vi "PID_position_radian.vi"() -> ()   [LabVIEW 2014]
uses:
  <vilib>/FPGAPlugInAG/cRIO-9068/niLvFpga_Open_cRIO-9068.vi
  <vilib>/rvi/interface/common/dynamic/niFpgaDynamicAddResources.vi
  <vilib>/Utility/error.llb/Error Cluster From Error Code.vi
  <vilib>/rvi/errors/niLvFpgaAdjustHostInterfaceError.vi
  <vilib>/addons/control/pid/pid.llb/PID (DBL).vi
  <vilib>/FPGAPlugInAG/Dynamic/niLvFpga_Close_Dynamic.vi
  <vilib>/rvi/interface/nirviOpenFPGA/nirviOpenFPGA.xnode
  FPGA Bitfiles/Motortest_FPGATarget_test6auto_Jx62XASY7Q8.lvbitx
  <vilib>/rvi/interface/nirviReadWriteControl/nirviReadWriteControl.xnode
  <vilib>/rvi/interface/nirviCloseFPGA/nirviCloseFPGA.xnode
  NiFpgaLv.dll
  <vilib>/rvi/interface/Simulation/niFpgaSimulationCallBeginRW.vi
  <vilib>/addons/control/pid/NI_PID_pid.lvlib
panel:
  in  "stop":bool
  out "Position [Round]":sgl
  out "Velocity [RPS]":sgl
  in  "PID Velocity":T1={"proportional gain (Kc)"=0.0006, "integral time (Ti, min)"=0.0005, "derivative time (Td, min)"=0.0} {"derivative time (Td, min)" format="%.4f"; "integral time (Ti, min)" format="%.4e"; "proportional gain (Kc)" format="%.4e"}
  in  "output range":cluster{"output high":dbl, "output low":dbl}={"output high"=1.0, "output low"=-1.0} {"output low" format="%.2f"; "output high" format="%.2f"}
  out "Velocity":sgl[](graph)
  out "Error":dbl(slide) scale=0.0..50.0
  out "Duty Cycle":dbl(slide) scale=0.0..1.0
  out "Duty Cycle 2":dbl[](graph)
  in  "Desired Position\n[Radian]":dbl=1500.0
  in  "PID Position":T1={"proportional gain (Kc)"=1.5, "integral time (Ti, min)"=0.0, "derivative time (Td, min)"=0.0} {"derivative time (Td, min)" format="%.3f"; "integral time (Ti, min)" format="%.3f"; "proportional gain (Kc)" format="%.3f"}
  out "Position":sgl[](graph)
  out "Velocity Setpoint":dbl[](graph)
  out "Velocity Setpoint [rad/second]":cluster{dbl[], dbl[]}(graph)
  out "Position [rad]":cluster{dbl[], sgl[]}(graph)
  out "Velocity [rad/second]":cluster{dbl[], sgl[]}(graph)
  out "Duty Cycle":cluster{dbl[], dbl[]}(graph)
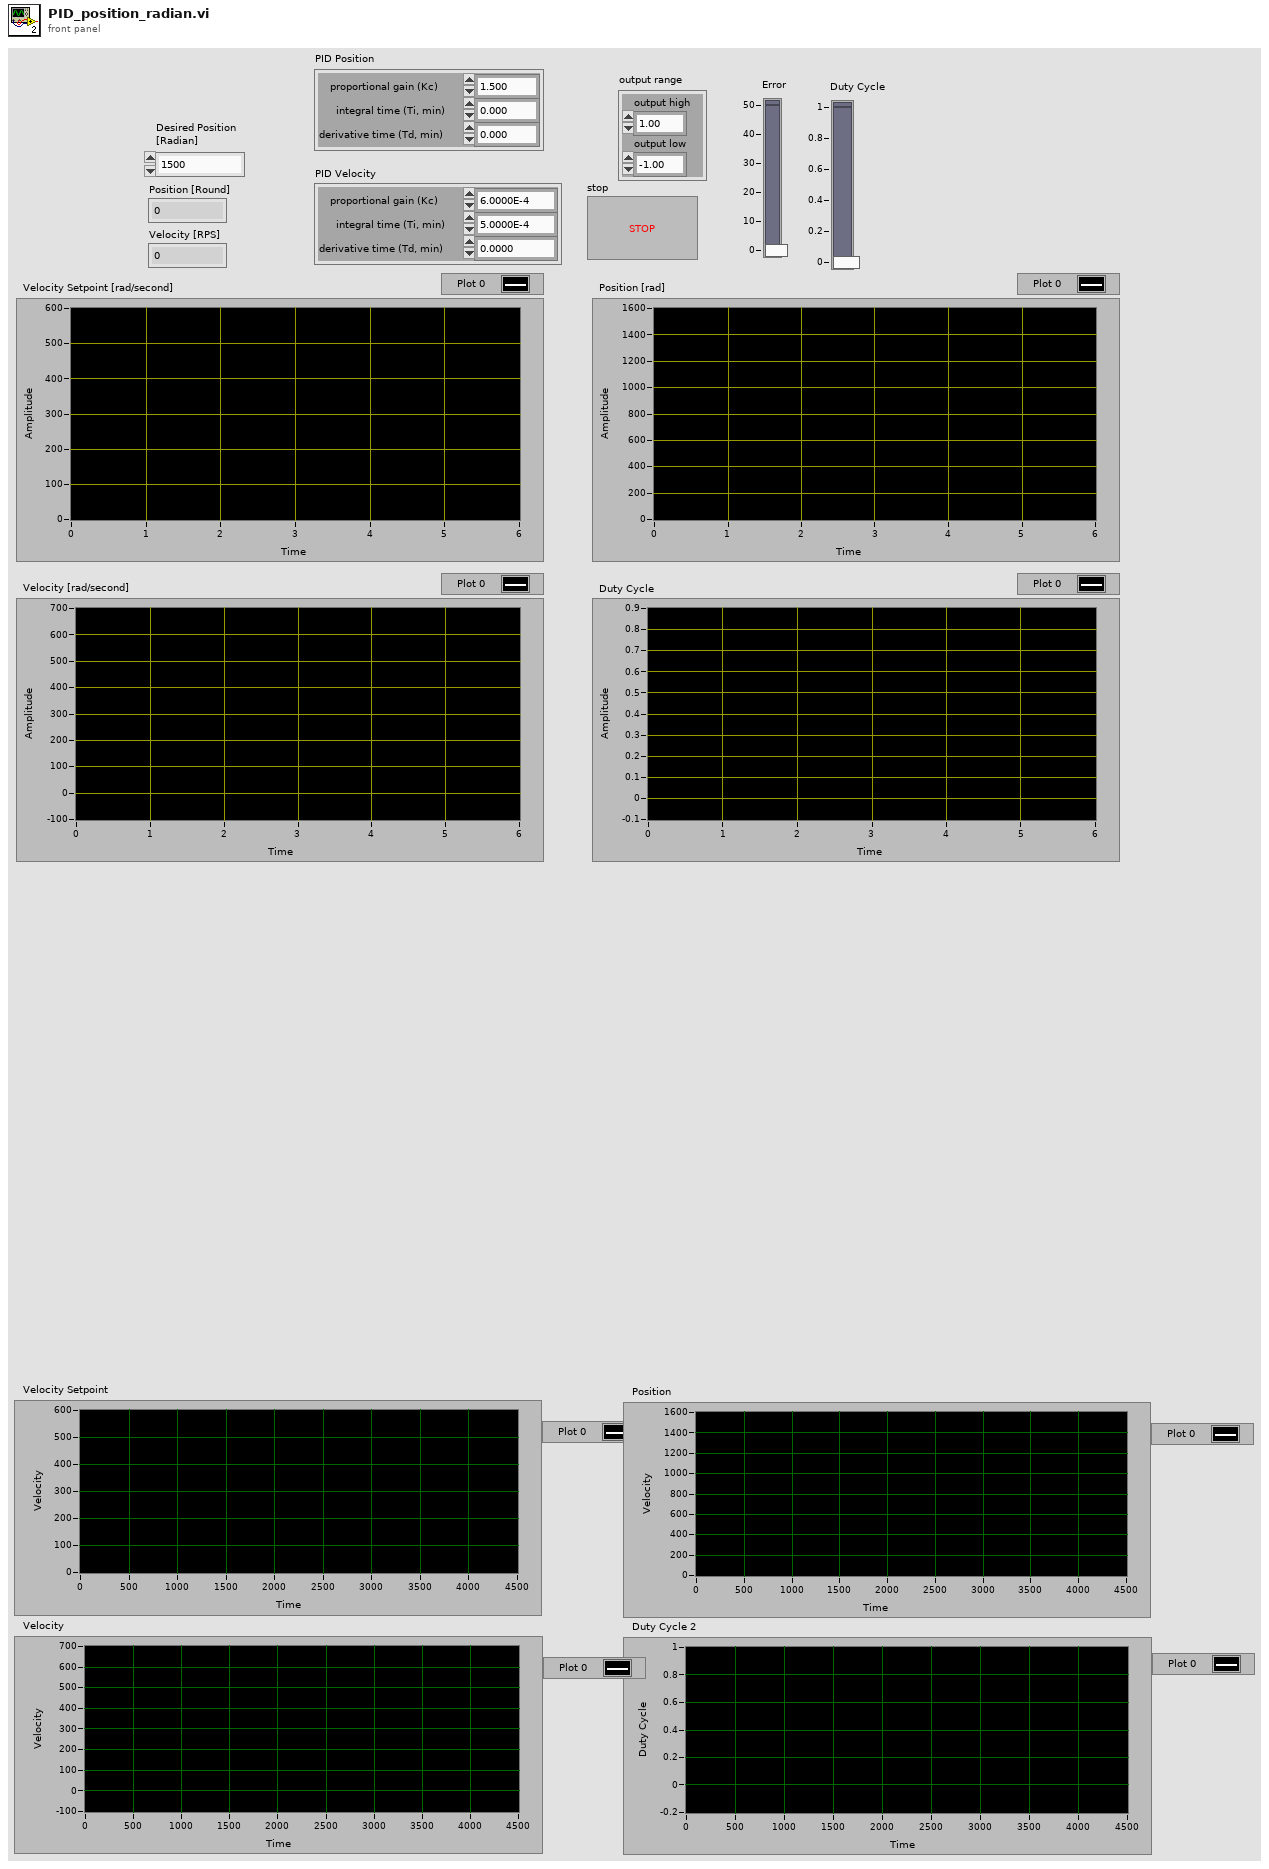
[diagram p1: front panel]
types:
  T1 = cluster{"proportional gain (Kc)":dbl, "integral time (Ti, min)":dbl, "derivative time (Td, min)":dbl}
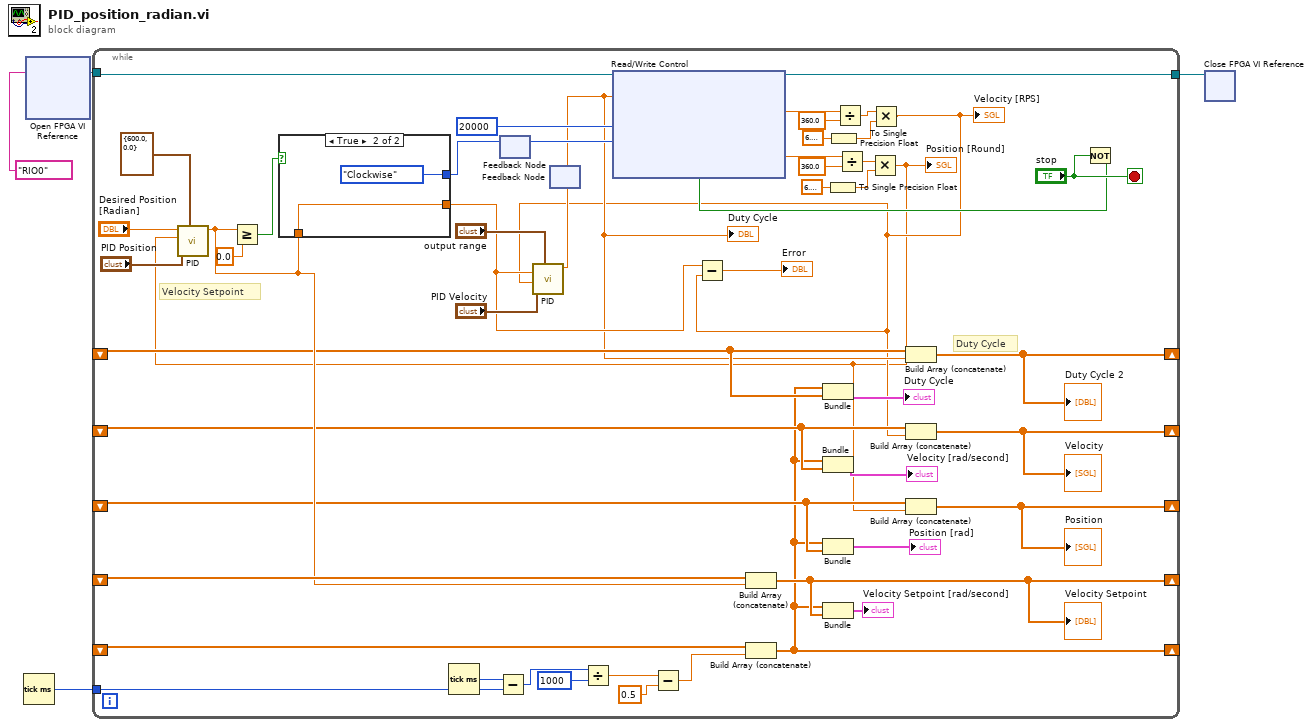
[diagram p0: block diagram]
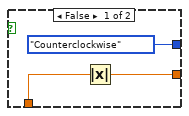
[diagram p2: hidden frame]
diagram:
  n1 = Tick Count (ms)() -> (millisecond timer value=w2:u32)
  n2 = xnode "Open FPGA VI Reference"("resource name"=tag "RIO0") -> ("FPGA VI Reference Out"=w1:refnum<k20>)  [unwired: 1 in, 1 out]
  n3 = while {
    tunnel: w1 -> [w56]
    tunnel: [w55] -> w4
    shift-right: [w43] -> _
    shift-left: _ -> [w19]
    shift-right: [w44] -> _
    shift-left: _ -> [w15]
    shift-right: [w38] -> _
    shift-left: _ -> [w18]
    shift-right: [w21] -> _
    shift-left: _ -> [w32]
    shift-right: [w14] -> _
    shift-left: _ -> [w30]
    tunnel: w2 -> [w28]
    stop <- "stop" stop-if-true
    # "Velocity Setpoint"
    # "Duty Cycle"
    n4 = Tick Count (ms)() -> (millisecond timer value=w27:u32)
    n5 = Subtract(x=w27, y=w28) -> (x-y=w26:u32)
    n6 = feedback #1() -> (w34:enum8{"Clockwise", "Counterclockwise"})  [unwired: 1 in]
    n7 = feedback #2() -> (w13:dbl)  [unwired: 1 in]
    "Duty Cycle" <- w13
    n8 = Divide(x=w26, y=u32 1000) -> (x/y=w24:dbl)
    n9 = Subtract(x=w24, y=0.5) -> (x-y=w25:dbl)
    n10 = Build Array (concatenate)(w30, w25) -> (w14:dbl[])
    n11 = Bundle(w14, w19) -> (→"Duty Cycle":cluster{dbl[], dbl[]})  [unwired: 1 in]
    n12 = Bundle(w14, w15) -> (→"Velocity [rad/second]":cluster{dbl[], sgl[]})  [unwired: 1 in]
    n13 = Bundle(w14, w18) -> (→"Position [rad]":cluster{dbl[], sgl[]})  [unwired: 1 in]
    n14 = To Single Precision Float(number=6.283185307179586 ("Pi Multiplied By 2")) -> (single precision float=w6:sgl)
    n15 = To Single Precision Float(number=6.283185307179586 ("Pi Multiplied By 2")) -> (single precision float=w10:sgl)
    n16 = Build Array (concatenate)(w19, w13) -> (w43:dbl[])
    "Duty Cycle 2" <- w43
    n17 = Not(x="stop") -> (.not. x?=w53:bool)
    n18 = xnode "Read/Write Control"("FPGA VI Reference In"=w56, "duty cycle (periods)"=w13, "Velocity Interval (uSec)"=u32 20000, "Mod1/Drive Direction"=w34, "Mod1/Motor"=w53) -> ("FPGA VI Reference Out"=w55:refnum<k20>, "Velocity (Degrees/Second)"=w46:sgl, "Position (Degrees)"=w49:sgl)  [unwired: 1 in, 1 out]
    n19 = Divide(x=w46, y=sgl 360.0) -> (x/y=w11:sgl)
    n20 = Divide(x=w49, y=sgl 360.0) -> (x/y=w7:sgl)
    n21 = Multiply(x=w7, y=w6) -> (x*y=w5:sgl)
    "Position [Round]" <- w5
    n22 = call-poly <vilib>:"PID.vi"("output range"=cluster{"output high":dbl, "output low":dbl} {"output high"=600.0, "output low"=0.0}, "PID gains"="PID Position", "process variable"=w5, "setpoint"="Desired Position\n[Radian]") -> ("output"=w31:dbl)  [unwired: 6 in, 1 out]
    n23 = Greater Or Equal?(x=w31, y=0.0) -> (x >= y?=w36:bool)
    n24 = case shown="True" w36 {
      tunnel: [enum8{"Clockwise", "Counterclockwise"}."Counterclockwise" ("Mod1/Drive Direction") enum8{"Clockwise", "Counterclockwise"}."Clockwise" ("Mod1/Drive Direction")] -> w35
      tunnel: w31 -> [w58 w60]
      tunnel: [w57 w60] -> w33
      frame False {
        n25 = Absolute Value(x=w58) -> (abs(x)=w57:dbl)
      }
      frame True {
      }
    }
    n26 = feedback-in #1(w35) -> ()
    n27 = Build Array (concatenate)(w32, w31) -> (w21:dbl[])
    "Velocity Setpoint" <- w21
    n28 = Bundle(w14, w21) -> (→"Velocity Setpoint [rad/second]":cluster{dbl[], dbl[]})  [unwired: 1 in]
    n29 = Multiply(x=w11, y=w10) -> (x*y=w9:sgl)
    "Velocity [RPS]" <- w9
    n30 = call-poly <vilib>:"PID.vi"("output range"="output range", "PID gains"="PID Velocity", "process variable"=w9, "setpoint"=w33) -> ("output"=w42:dbl)  [unwired: 6 in, 1 out]
    n31 = feedback-in #2(w42) -> ()
    n32 = Subtract(x=w33, y=w9) -> (x-y=→"Error":dbl)
    n33 = Build Array (concatenate)(w15, w9) -> (w44:sgl[])
    "Velocity" <- w44
    n34 = Build Array (concatenate)(w18, w5) -> (w38:sgl[])
    "Position" <- w38
  }
  n35 = xnode "Close FPGA VI Reference"("FPGA VI Reference In"=w4) -> ()  [unwired: 1 in, 1 out]
